vi "ArmSetXYZDemand.vi"(9 "SetZ":dbl, 10 "SetY":dbl, 11 "SetX":dbl) -> ()   [LabVIEW 2020]
doc: "Set XYZ demand for X,Y,Z arm globals and for ArmXYZToR-L-E, and set those outputs to ArmSetDemands\n\nInputs:\n--SetX--Double\n--SetY--Double\n--SetZ--Double"
uses:
  ArmGlobal.vi
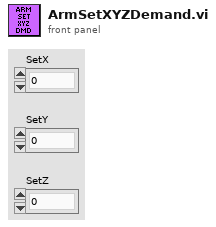
[diagram p1: front panel]
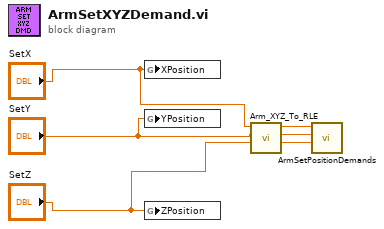
[diagram p0: block diagram]
diagram:
  n1 = global write "ArmGlobal.vi" "XPosition"("SetX") -> ()
  n2 = global write "ArmGlobal.vi" "YPosition"("SetY") -> ()
  n3 = global write "ArmGlobal.vi" "ZPosition"("SetZ") -> ()
  n4 = call "Arm_XYZ_To_RLE.vi"("Z"="SetZ", "Y"="SetY", "X"="SetX") -> ("Extend"=w1:dbl, "Lift"=w2:dbl, "Rotate"=w3:dbl)  [unwired: 6 in]
  n5 = call "ArmSetPositionDemands.vi"("SetExtendPositonDemand(in)"=w1, "SetLIftPostionDemand(d)"=w2, "SetRotatePostionDemand(d)"=w3) -> ()  [unwired: 9 in]
